vi "Register Verbose Explanation.vi"(8 "error in (no error)":errorcluster, 9 "Explanation":string, 10 "Unique ID":string, 11 "Test Manager in":refnum<class "Test Manager.lvclass">=refnum) -> (0 "error out":errorcluster, 3 "Test Manager out":refnum<class "Test Manager.lvclass">)   [LabVIEW 2020, in "Caraya.lvlib" / "Test Manager.lvclass"]
uses:
  Test Manager.lvclass
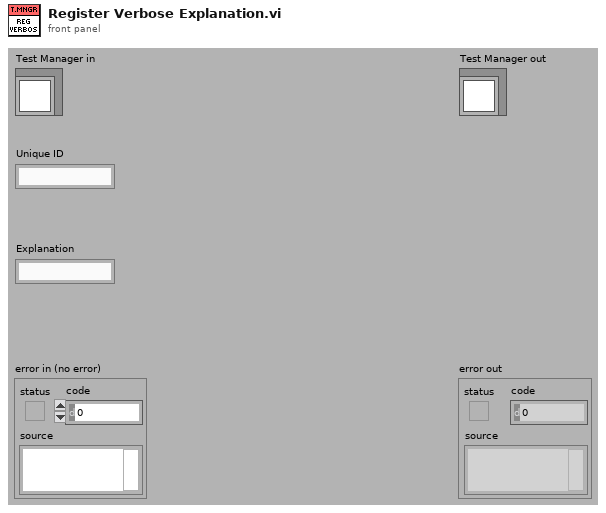
[diagram p1: front panel]
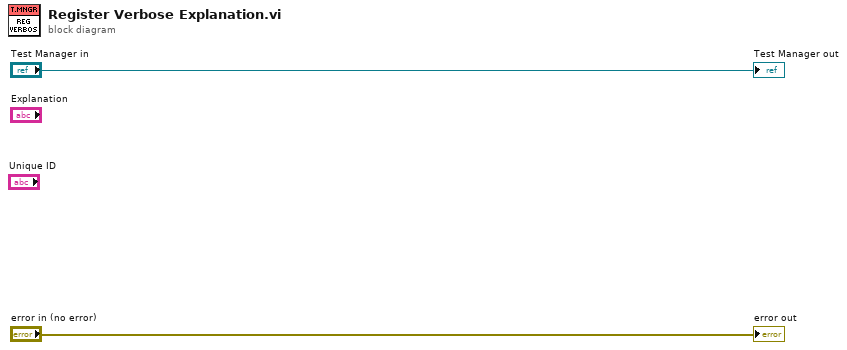
[diagram p0: block diagram]
diagram:
  "error out" <- "error in (no error)"
  "Test Manager out" <- "Test Manager in"
